vi "GDSAPI_Example_CreateClass.vi"() -> ()   [LabVIEW 2020]
uses:
  GDSAPI_SubVIs/GDSAPI_ProjectIconType.ctl
  GDSAPI_SubVIs/GDSAPI_ClassProviderType.ctl
  ClassProviders/Common/ScriptingFunctions/Scripting_ConnectorPanePatternType.ctl
  GDSAPI_CreateClassType.ctl
  GDSAPI_SubVIs/GDSAPI_ClassTemplateType.ctl
panel:
  out "VIs Loaded into memory":string[](array[string])
  in  "Stop(hidden)":bool
  out "error out":errorcluster
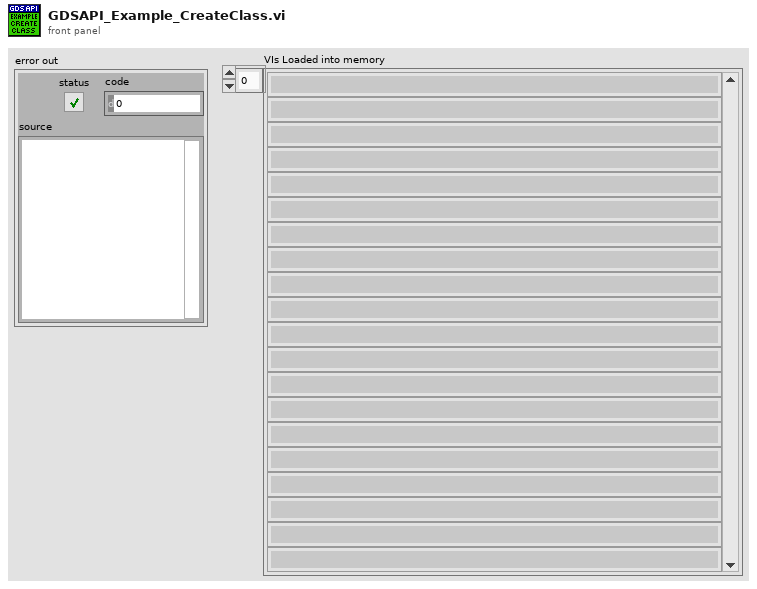
[diagram p1: front panel]
types:
  T1 = typedef "Scripting_ConnectorPanePatternType.ctl" = u16
  T2 = typedef "GDSAPI_ClassProviderType.ctl" = enum16{"LabVIEW Native(By value)", "GOOP-3(By reference)", "GOOP-4(By reference)"}
  T3 = typedef "GDSAPI_ProjectIconType.ctl" = enum16{"BlueCircle", "BlueFrame", "BlueFull", "BlueMessage", "BrownCircle", "BrownFrame", "BrownFull", "BurgundyCircle", "BurgundyFrame", "BurgundyFull", "CyanCircle", "CyanFrame", "CyanFull", "DarkBlueCircle", "DarkBlueFrame", "DarkBlueFull", "ForestGreenCircle", "ForestGreenFrame", "ForestGreenFull", "GrayCircle", "GrayFrame", "GrayFull", "GreenCircle", "GreenFrame", "GreenFull", "Interface", "InterfaceBlue", "InterfaceBrown", "InterfaceBurgundy", "InterfaceCyan", "InterfaceDarkBlue", "InterfaceForestGreen", "InterfaceGray", "InterfaceGreen", "InterfaceLightGreen", "InterfaceLightRed", "InterfacePink", "InterfacePurple", "InterfaceRed", "InterfaceYellow", "LightGreenCircle", "LightGreenFrame", "LightGreenFull", "LightRedCircle", "LightRedFrame", "LightRedFull", "PinkCircle", "PinkFrame", "PinkFull", "PurpleCircle", "PurpleFrame", "PurpleFull", "RedCircle", "RedFrame", "RedFull", "YellowCircle", "YellowFrame", "YellowFull"}
  T4 = typedef "GOOP_WireConfigurationType.ctl" = cluster{"Edge thickness":i32, "Edge color":u32, "Center thickness":i32, "Center pattern":T5, "CenterColor1":u32, "CenterColor2":u32, "Tunnels and terminals colors":u32}
  T5 = typedef "GOOP_WirePattern.ctl" = enum16{"Solid", "Large dash", "Small dash"}
  T6 = typedef "GDSAPI_CreateClassType.ctl" = cluster{"ClassProvider":T2, "NewClassFolder":path, "ParentLvClassFilePath":path, "ClassName":string, "ClassDescription":string, "ClassTemplate":T7, "ParentInterfacesFilePath":path[]}
  T7 = typedef "GDSAPI_ClassTemplateType.ctl" = enum16{"Standard", "Singleton", "Interface(By Aggregation)", "Interface(By VI Server)"}
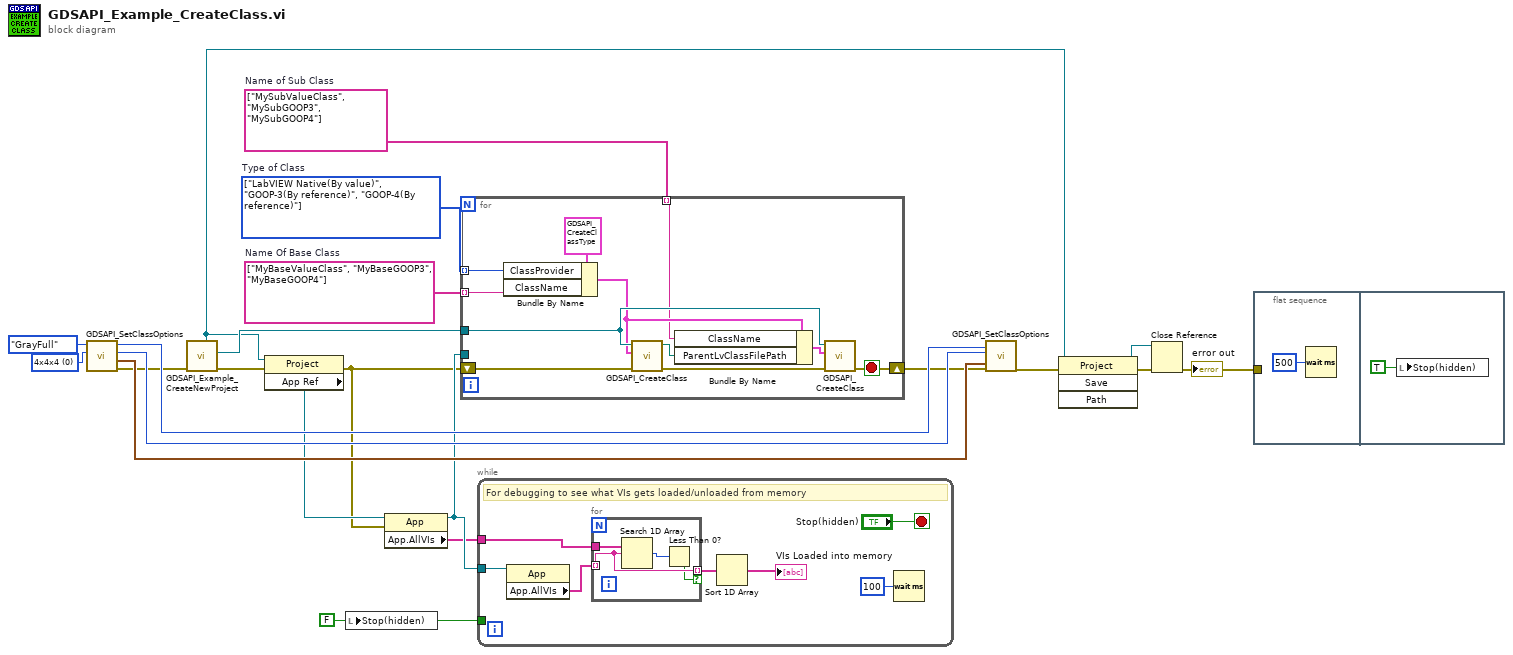
[diagram p0: block diagram]
diagram:
  w6 = T1 0 items=["4x4x4", "5x6x5", "6x8x6"] ("PatternIn")
  w8 = FALSE ("stop")
  w12 = string[] ["MySubValueClass", "MySubGOOP3", "MySubGOOP4"]  # Name of Sub Class
  w4 = string[] ["MyBaseValueClass", "MyBaseGOOP3", "MyBaseGOOP4"]  # Name Of Base Class
  w5 = T2[] [enum."LabVIEW Native(By value)", enum."GOOP-3(By reference)", enum."GOOP-4(By reference)"] items=["LabVIEW Native(By value)", "GOOP-3(By reference)", "GOOP-4(By reference)"]  # Type of Class
  n1 = call "GDSAPI_SetClassOptions.vi"("PatternIn"=w6, "ProjectIconType"=GDSAPI_ProjectIconType."GrayFull") -> ("error out"=w18:errorcluster, "WireConfiguration-Before"=w19:T4, "Pattern-Before"=w20:T1, "ProjectIcon-Before"=w21:T3)  [unwired: 6 in]
  n2 = call "GDSAPI_Example_CreateNewProject.vi"("error in (no error)"=w18) -> ("error out"=w3:errorcluster, "ProjectItem out"=w17:refnum<vi>, "ProjectRefOut"=w11:refnum<vi>)  [unwired: 7 in, 1 out]
  n3 = property class="Project"(reference=w11, error in=w3) -> (error out=w2:errorcluster, "App Ref"=w10:refnum<vi>)  [unwired: 1 out]
  n4 = local write "Stop(hidden)"(w8) -> ()
  n5 = property class="App"(reference=w10, error in=w2) -> (reference out=w9:refnum<vi>, "App.AllVIs"=w7:string[])  [unwired: 1 out]
  n6 = for {
    tunnel: w17 -> [w33]
    tunnel: w12 -> [w29] mode=indexing
    tunnel: w4 -> [w28] mode=indexing
    tunnel: w5 -> [w27] mode=indexing
    shift-right: [w26] -> w16
    shift-left: w2 -> [w24]
    tunnel: w9 -> [_]
    stop <- w26 stop-if-true
    n7 = Bundle By Name(cluster=T6 {"ClassProvider"=enum."LabVIEW Native(By value)", "NewClassFolder"=path "", "ParentLvClassFilePath"=path "", "ClassName"="", "ClassDescription"="", "ClassTemplate"=enum."Standard", "ParentInterfacesFilePath"=[]} ("CreateClassType"), "ClassProvider"=w27, "ClassName"=w28) -> (w30:T6)
    n8 = call "GDSAPI_CreateClass.vi"("error in (no error)"=w24, "CreateClassType"=w30, "ProjectItemToCreateClassUnder"=w33) -> ("error out"=w25:errorcluster, "LvClassFileOut"=w32:path)  [unwired: 6 in, 1 out]
    n9 = Bundle By Name(cluster=w30, "ClassName"=w29, "ParentLvClassFilePath"=w32) -> (w31:T6)
    n10 = call "GDSAPI_CreateClass.vi"("error in (no error)"=w25, "CreateClassType"=w31, "ProjectItemToCreateClassUnder"=w33) -> ("error out"=w26:errorcluster)  [unwired: 6 in, 2 out]
  }
  n11 = while {
    tunnel: w9 -> [w37]
    tunnel: w8 -> [_]
    tunnel: w7 -> [w34]
    stop <- "Stop(hidden)" stop-if-true
    # "For debugging to see what VIs gets loaded/unloaded from memory"
    n12 = property class="App"(reference=w37) -> ("App.AllVIs"=w36:string[])  [unwired: 1 in, 2 out]
    n13 = for {
      tunnel: w36 -> [w42] mode=indexing
      tunnel: w34 -> [w44]
      tunnel: [w42] -> w39 mode=indexing if=w41
      n14 = Search 1D Array(1D array=w44, element=w42) -> (index of element=w43:i32)  [unwired: 1 in]
      n15 = Less Than 0?(x=w43) -> (x < 0?=w41:bool)
    }
    n16 = Sort 1D Array(array=w39) -> (sorted array=→"VIs Loaded into memory":string[])
    n17 = Wait (ms)(milliseconds to wait=u32 100) -> ()  [unwired: 1 out]
  }
  n18 = call "GDSAPI_SetClassOptions.vi"("error in (no error)"=w16, "WireConfiguration"=w19, "PatternIn"=w20, "ProjectIconType"=w21) -> ("error out"=w15:errorcluster)  [unwired: 4 in, 3 out]
  n19 = invoke class="Project" method="Save"(reference=w11, error in=w15) -> (reference out=w13:refnum<vi>, error out=w14:errorcluster)  [unwired: 2 in, 2 out]
  n20 = Close Reference(reference=w13, error in (no error)=w14) -> (error out=w1:errorcluster)
  "error out" <- w1
  n21 = flat-sequence {
    tunnel: w1 -> [_]
    frame #0 {
      n22 = Wait (ms)(milliseconds to wait=u32 500) -> ()  [unwired: 1 out]
    }
    frame #1 {
      n23 = local write "Stop(hidden)"(TRUE ("stop")) -> ()
    }
  }
